vi "Initialize DB.vi"(8 "error in (no error)":errorcluster) -> (0 "error out":errorcluster, 2 "DB Connected?":bool, 3 "Db Path":string)   [LabVIEW 2024]
uses:
  Variables/Download Confrigurations.vi
  <vilib>/addons/database/Connection.llb/DB Tools Open Connec (Path).vi
  <vilib>/addons/database/NI_Database_API.lvlib
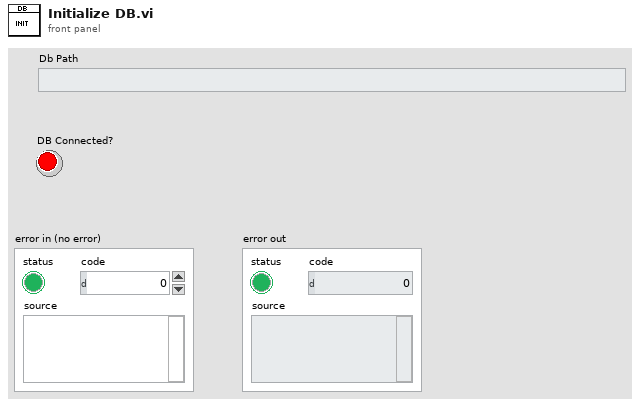
[diagram p1: front panel]
types:
  T1 = typedef "NI_Database_API.lvlib/Conn ObjectReference.ctl" = refnum<k1>
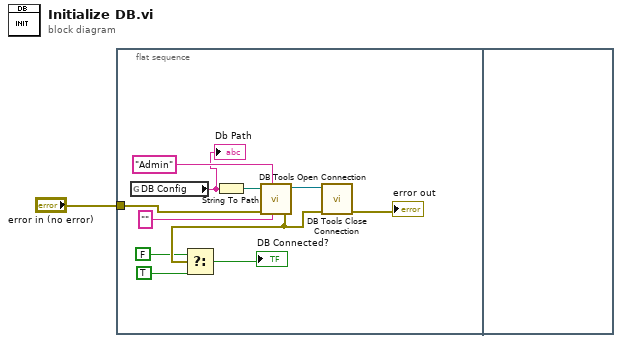
[diagram p0: block diagram]
diagram:
  n1 = flat-sequence {
    tunnel: "error in (no error)" -> [w8]
    frame #0 {
      n2 = global read "Download Confrigurations.vi" "DB Config"() -> (w10:string)
      "Db Path" <- w10
      n3 = String To Path(string=w10) -> (path=w12:path)
      n4 = call-poly <vilib>:"DB Tools Open Connection.vi"("password"="", "userID"="Admin", "error in (no error)"=w8, "connection information"=w12) -> ("error out"=w6:errorcluster, "connection reference"=w7:T1)  [unwired: 4 in]
      n5 = Select(t=FALSE, s=w6, f=TRUE) -> (s? t:f=→"DB Connected?":bool)
      n6 = call <vilib>:"DB Tools Close Connection.vi"("error in (no error)"=w6, "connection reference"=w7) -> ("error out"=→"error out":errorcluster)  [unwired: 5 in]
    }
    frame #1 {
    }
  }
